vi "Read moduleName.vi"(8 "error in (no error)":errorcluster, 11 "Enumeration in":refnum<class "Enumeration.lvclass">) -> (0 "error out":errorcluster, 2 "moduleName":string, 3 "Enumeration out":refnum<class "Enumeration.lvclass">)   [LabVIEW 2016, in "Enumeration.lvclass"]
uses:
  Enumeration.lvclass
  Enumeration.lvclass/Enumeration.ctl
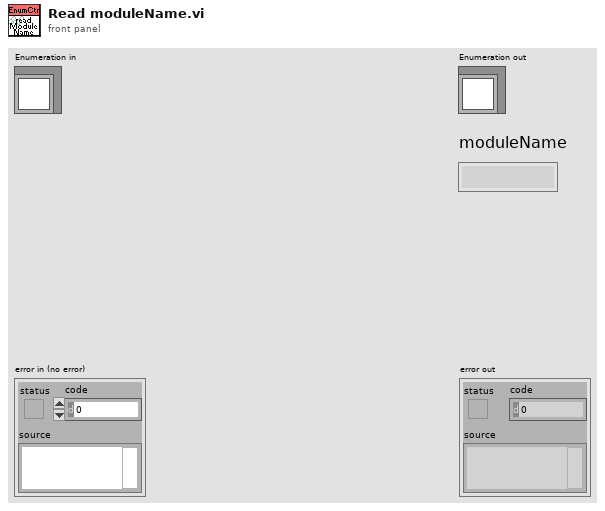
[diagram p1: front panel]
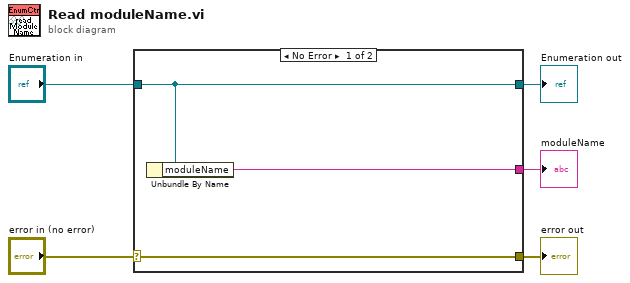
[diagram p0: block diagram]
diagram:
  n1 = case shown="No Error" "error in (no error)" {
    selector: "error in (no error)" -> [w8 w9]
    tunnel: [w8 w9] -> w4
    tunnel: [w7 w10] -> w2
    tunnel: "Enumeration in" -> [w7 w10]
    tunnel: [w6 _] -> w1
    frame No Error {
      n2 = Unbundle By Name(w7) -> ("moduleName"=w6:string)
    }
    frame Error {
    }
  }
  "error out" <- w4
  "Enumeration out" <- w2
  "moduleName" <- w1
